vi "ClassAttributes_ReadWriteClassAttributes_4x4x4.vi"(8 "error in (no error)":errorcluster, 11 "reference in":refnum<class>) -> (0 "error out":errorcluster, 3 "reference out":refnum<class>)   [LabVIEW 2020]
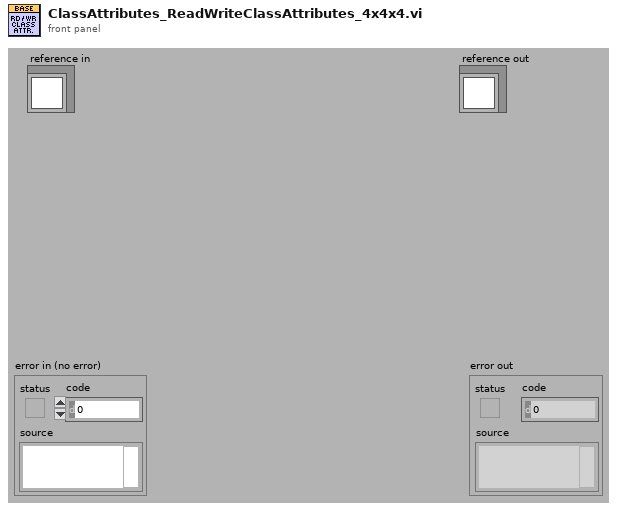
[diagram p1: front panel]
types:
  T1 = typedef "ClassAttributes_ClassAttributes.ctl" = cluster{"classAttribute1":bool}
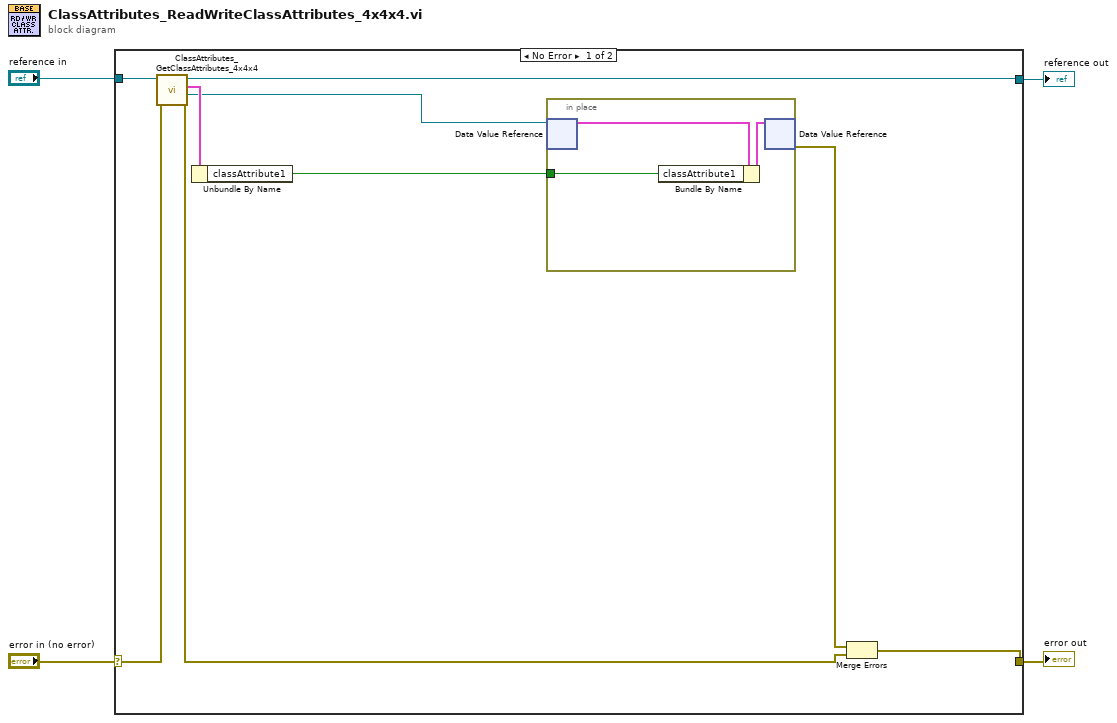
[diagram p0: block diagram]
diagram:
  n1 = case shown="No Error" "error in (no error)" {
    selector: "error in (no error)" -> [w12 w18]
    tunnel: [w6 w18] -> w3
    tunnel: [w5 w17] -> w1
    tunnel: "reference in" -> [w13 w17]
    frame No Error {
      n2 = call "ClassAttributes_GetClassAttributes_4x4x4.vi"("error in"=w12, "reference in"=w13) -> ("error out"=w7:errorcluster, "Class attribute Reference"=w9:refnum<data-value>, "Class attribute"=w11:T1, "reference out"=w5:refnum<class>)  [unwired: 6 in]
      n3 = Unbundle By Name(w11) -> ("classAttribute1"=w8:bool)
      n4 = in-place {
        in-place-border: w8 -> [w16]
        n5 = in-place-dvr #1(w9) -> (w15:T1)  [unwired: 1 out]
        n6 = Bundle By Name(cluster=w15, "classAttribute1"=w16) -> (w14:T1)
        n7 = in-place-dvr #1(w14) -> (w10:errorcluster)  [unwired: 1 out]
      }
      n8 = Merge Errors(w10, w7) -> (w6:errorcluster)
    }
    frame Error {
    }
  }
  "error out" <- w3
  "reference out" <- w1
